vi "GRNF_POT.vi"(7 "RefNum Name":string="My Motor RefNum") -> (0 "Error":errorcluster, 3 "Device Reference":T1={"DevStatus"={"status"=FALSE, "code"=0, "source"=""}, "Analog Channel"=enum."Invalid", "Invert Output"=FALSE})   [LabVIEW 2019]
uses:
  <vilib>/Rock Robotics/WPI/Potentiometer/WPI_PotentiometerDevRef.ctl
  <vilib>/Rock Robotics/SystemInterfaces/AI/FPGA_AIChannel.ctl
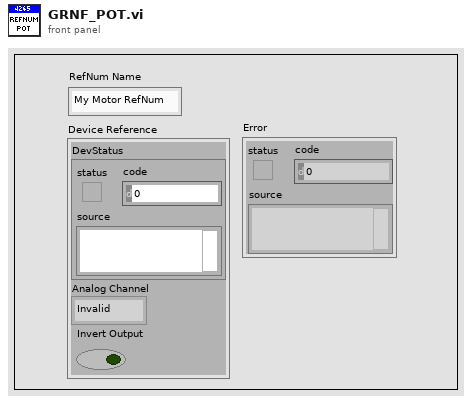
[diagram p1: front panel]
types:
  T1 = typedef "WPI_PotentiometerDevRef.ctl" = cluster{"DevStatus":errorcluster, "Analog Channel":T2, "Invert Output":bool}
  T2 = typedef "FPGA_AIChannel.ctl" = enum8{"AI 0", "AI 1", "AI 2", "AI 3", "AI MXP 0", "AI MXP 1", "AI MXP 2", "AI MXP 3", "Invalid"}
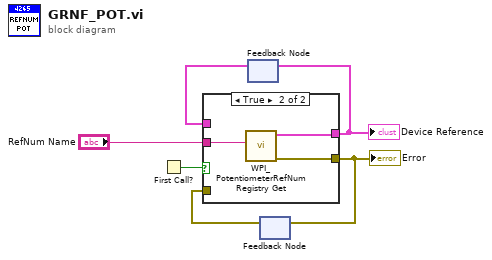
[diagram p0: block diagram]
diagram:
  n1 = First Call?() -> (First Call?: T/F=w6:bool)
  n2 = feedback #1() -> (w5:T1)  [unwired: 1 in]
  n3 = feedback #2() -> (w1:errorcluster)  [unwired: 1 in]
  n4 = case shown="True" w6 {
    tunnel: [w8 w10] -> w4
    tunnel: w5 -> [w8 _]
    tunnel: "RefNum Name" -> [_ w11]
    tunnel: [w7 w9] -> w2
    tunnel: w1 -> [w7 _]
    frame False {
    }
    frame True {
      n5 = call <vilib>:"WPI_PotentiometerRefNum Registry Get.vi"("refnum name"=w11) -> ("error out"=w9:errorcluster, "PotDevRef"=w10:T1)  [unwired: 9 in]
    }
  }
  "Device Reference" <- w4
  "Error" <- w2
  n6 = feedback-in #1(w4) -> ()
  n7 = feedback-in #2(w2) -> ()
